vi "LWXPS_GatheringExternalDataGet.vi"(0 "XPS Reference IN":refnum<k24>, 5 "Index Point":i32, 11 "LabVIEW error IN":errorcluster) -> (4 "XPS Reference OUT":refnum<k24>, 6 "Returned error code":i32, 8 "Data Buffer Line":string, 10 "XPS Error String":string, 15 "LabVIEW error OUT":errorcluster)   [LabVIEW 2014]
uses:
  D:/XPSQ8_LabView_Library/Development/Source/Dll/Newport.XPS.CommandInterface.dll
  Dll/Newport.XPS.CommandInterface.dll
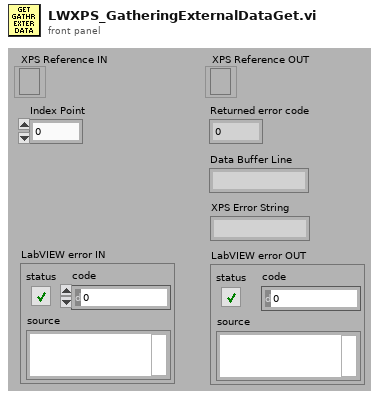
[diagram p1: front panel]
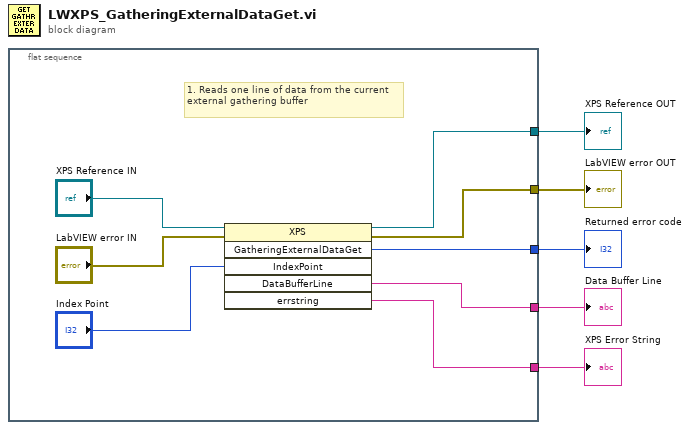
[diagram p0: block diagram]
diagram:
  n1 = flat-sequence {
    tunnel: [w12] -> w5
    tunnel: [w11] -> w4
    tunnel: [w10] -> w3
    tunnel: [w7] -> w1
    tunnel: [w8] -> w2
    frame #0 {
      # "1. Reads one line of data from the current external gathering buffer"
      n2 = invoke class="XPS" method="GatheringExternalDataGet"(reference="XPS Reference IN", error in="LabVIEW error IN", "IndexPoint"="Index Point") -> (reference out=w12:refnum<k24>, error out=w11:errorcluster, "GatheringExternalDataGet"=w10:i32, "DataBufferLine"=w7:string, "errstring"=w8:string)  [unwired: 3 in, 1 out]
    }
  }
  "XPS Reference OUT" <- w5
  "LabVIEW error OUT" <- w4
  "Returned error code" <- w3
  "XPS Error String" <- w2
  "Data Buffer Line" <- w1
